vi "BasicWrite.vi"   [LabVIEW 2020]
types:
  T1 = enum16{"open", "replace", "create", "open or create", "replace or create", "replace or create with confirmation"}
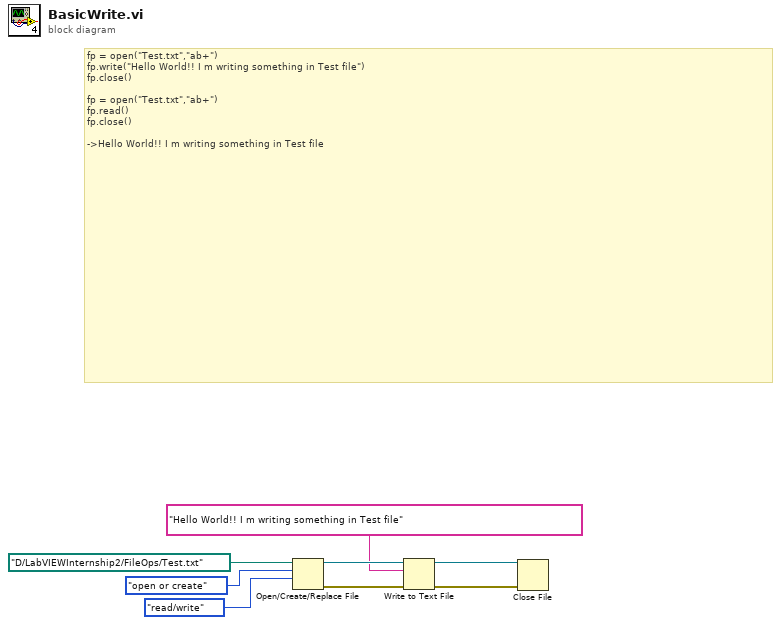
[diagram p0: block diagram]
diagram:
  # "fp = open(\"Test.txt\",\"ab+\")\nfp.write(\"Hello World!! I m writing something in Test file\")\nfp.close()\n\nfp = open(\"Test.txt\",\"ab+\")\nfp.read()\nfp.close()\n\n->Hello World!! I m writing something in Test file"
  n1 = Open/Create/Replace File(file path (use dialog)=path "D:/LabVIEWInternship2/FileOps/Test.txt", operation (0:open)=T1."open or create", access (0:read/write)=enum16{"read/write", "read-only", "write-only"}."read/write") -> (refnum out=w5:refnum<file>, error out=w4:errorcluster)  [unwired: 3 in, 1 out]
  n2 = Write to Text File(file (use dialog)=w5, text="Hello World!! I m writing something in Test file", error in=w4) -> (refnum out=w3:refnum<file>, error out=w2:errorcluster)  [unwired: 1 in, 1 out]
  n3 = Close File(refnum=w3, error in=w2) -> ()  [unwired: 2 out]
